vi "YAML.Multiline.vi"(2 "Key":string, 3 "Multiline":string) -> (1 "Output":string)   [LabVIEW 2016, in "AFM Control.lvclass"]
uses:
  AFM Control.lvclass
panel:
  # "This entire block of text will be the value of the 'literal_block' key,\n    with line breaks being preserved.\n\n    The literal continues until de-dented, and the leading indentation is\n    stripped.\n\n        Any lines that are 'more-indented' keep the rest of their indentation -\n        these lines will be indented by 4 spaces."
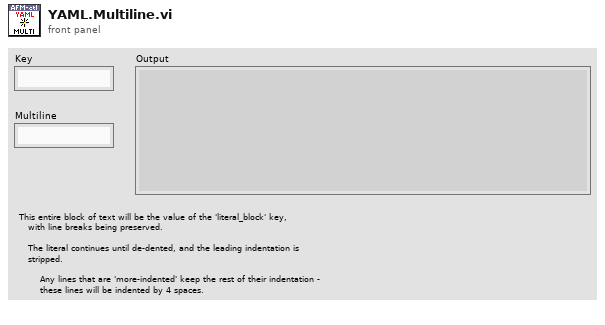
[diagram p1: front panel]
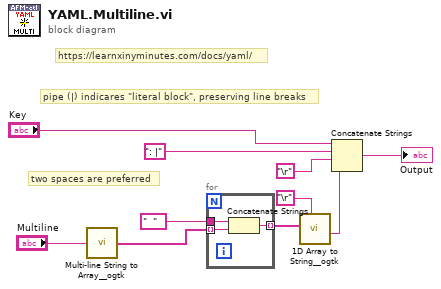
[diagram p0: block diagram]
diagram:
  # "pipe (|) indicares \"literal block\", preserving line breaks"
  # "two spaces are preferred"
  # "https://learnxinyminutes.com/docs/yaml/"
  n1 = call <userlib>:"Multi-line String to Array__ogtk.vi"("string"="Multiline") -> ("lines"=w3:string[])
  n2 = for {
    tunnel: w3 -> [w13] mode=indexing
    tunnel: "  " ("string") -> [w11]
    tunnel: [w12] -> w6 mode=indexing
    n3 = Concatenate Strings(w11, w13) -> (w12:string)
  }
  n4 = call <userlib>:"1D Array to String__ogtk.vi"("delimiter (Tab)"="\r", "Array of Strings"=w6) -> ("delimited string"=w8:string)  [unwired: 9 in]
  n5 = Concatenate Strings("Key", ": |" ("string"), "\r", w8) -> (→"Output":string)
